vi "DateFromSN.vi"(11 "SN":string) -> (3 "Date de fab":string)   [LabVIEW 2020]
panel:
  out "unsigned byte array":u8[](array[numeric])
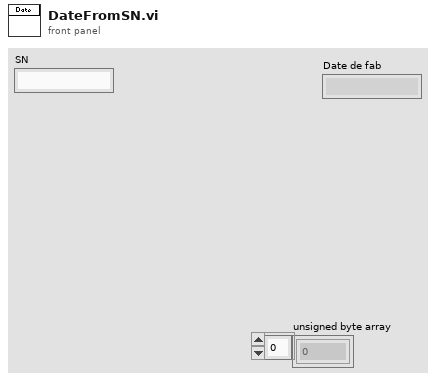
[diagram p1: front panel]
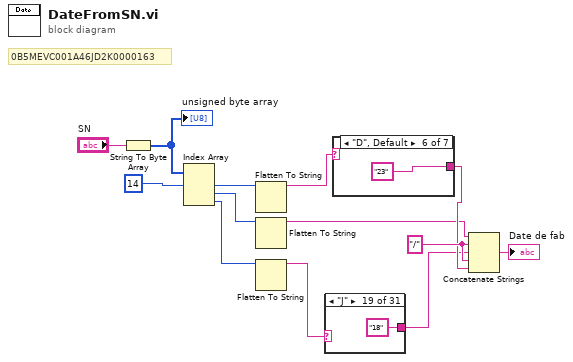
[diagram p0: block diagram]
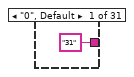
[diagram p2: hidden frame]
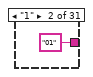
[diagram p3: hidden frame]
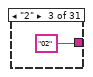
[diagram p4: hidden frame]
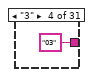
[diagram p5: hidden frame]
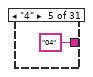
[diagram p6: hidden frame]
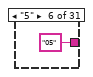
[diagram p7: hidden frame]
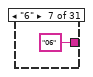
[diagram p8: hidden frame]
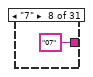
[diagram p9: hidden frame]
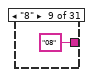
[diagram p10: hidden frame]
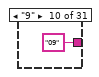
[diagram p11: hidden frame]
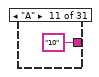
[diagram p12: hidden frame]
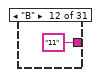
[diagram p13: hidden frame]
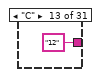
[diagram p14: hidden frame]
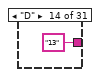
[diagram p15: hidden frame]
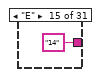
[diagram p16: hidden frame]
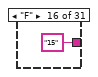
[diagram p17: hidden frame]
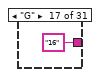
[diagram p18: hidden frame]
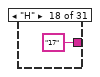
[diagram p19: hidden frame]
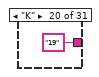
[diagram p20: hidden frame]
diagram:
  w7 = "/" ("string")
  # "0B5MEVC001A46JD2K0000163"
  n1 = String To Byte Array(string="SN") -> (unsigned byte array=w13:u8[])
  "unsigned byte array" <- w13
  n2 = Index Array(array=w13, index #1=14 ("index")) -> (element #1=w11:u8, element #2=w10:u8, element #3=w9:u8)  [unwired: 2 in]
  n3 = Flatten To String(anything=w11) -> (data string=w8:string)  [unwired: 3 in, 2 out]
  n4 = Flatten To String(anything=w10) -> (data string=w2:string)  [unwired: 3 in, 2 out]
  n5 = Flatten To String(anything=w9) -> (data string=w4:string)  [unwired: 3 in, 2 out]
  n6 = case shown="\"J\"" w4 {
    tunnel: ["31" "01" "02" "03" "04" "05" "06" "07" "08" "09" "10" "11" "12" "13" "14" "15" "16" "17" "18" "19" "20" "21" "22" "23" "24" "25" "26" "27" "28" "29" "30"] -> w1
    frame "0", Default {
    }
    frame "1" {
    }
    frame "2" {
    }
    frame "3" {
    }
    frame "4" {
    }
    frame "5" {
    }
    frame "6" {
    }
    frame "7" {
    }
    frame "8" {
    }
    frame "9" {
    }
    frame "A" {
    }
    frame "B" {
    }
    frame "C" {
    }
    frame "D" {
    }
    frame "E" {
    }
    frame "F" {
    }
    frame "G" {
    }
    frame "H" {
    }
    frame "J" {
    }
    frame "K" {
    }
    frame "L" {
    }
    frame "M" {
    }
    frame "N" {
    }
    frame "P" {
    }
    frame "R" {
    }
    frame "S" {
    }
    frame "T" {
    }
    frame "V" {
    }
    frame "W" {
    }
    frame "X" {
    }
    frame "Y" {
    }
  }
  n7 = case shown="\"D\", Default" w8 {
    tunnel: ["2018" "2019" "2020" "2021" "2022" "23" "2024"] -> w6
    frame "8" {
    }
    frame "9 " {
    }
    frame "A" {
    }
    frame "B" {
    }
    frame "C" {
    }
    frame "D", Default {
    }
    frame "E" {
    }
  }
  n8 = Concatenate Strings(w2, w7, w1, w7, w6) -> (→"Date de fab":string)
